vi "SettleDrift_v2.vi"() -> ()   [LabVIEW 2014]
uses:
  shared/CorrelImages (SubVI)Single.vi
  <userlib>/Nanonis Prog Interface V5/Nanonis Prog Interface.lvlib
panel:
  in  "stop":bool
  out "x drift":sgl format="%#_6p"
  out "y drift":sgl format="%#_6p"
  out "y Drift":sgl(graph)
  out "X Drift":sgl(graph)
  in  "Drift correction Pixels":i32=256
  in  "Img Current":sgl=2.5e-11 format="%#_6p"
  in  "Img Bias (V)":sgl=0.02 format="%_2p"
  in  "Img Speed":sgl=3e-08 format="%#_6p"
  in  "Channel index (0-23)":u8(ring) items=["Current"=0, "Z (m)"=14]
  # "Turn continuous scan off"
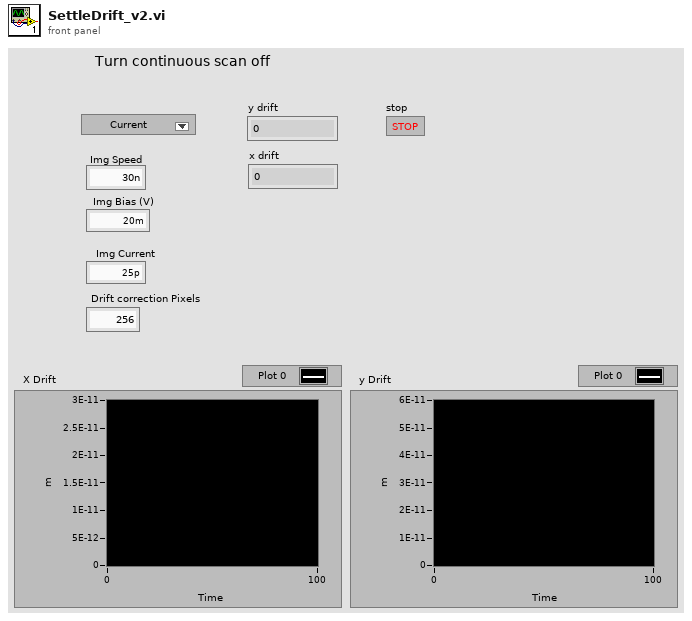
[diagram p1: front panel]
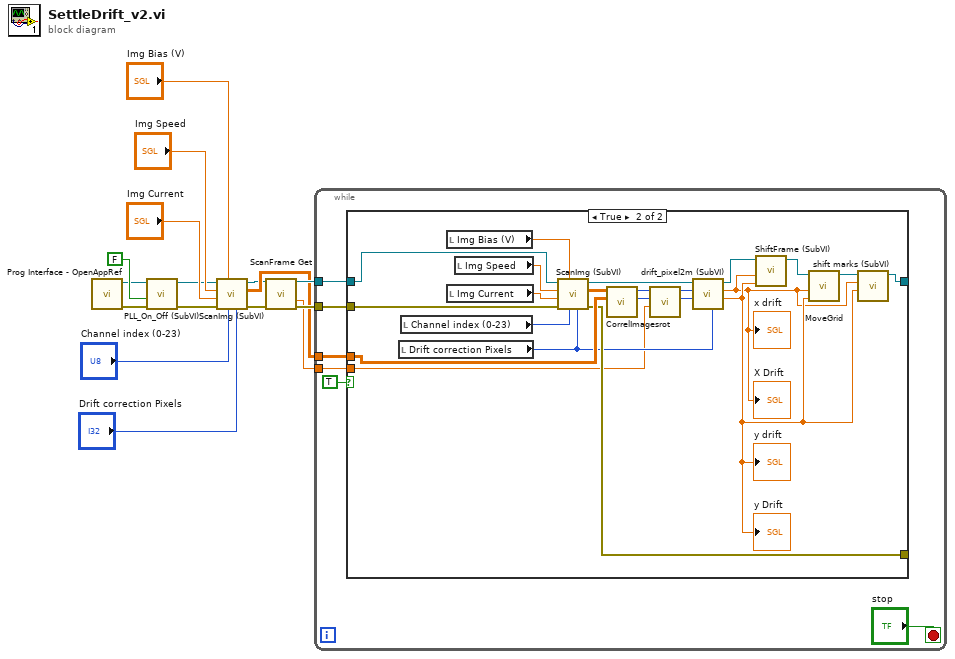
[diagram p0: block diagram]
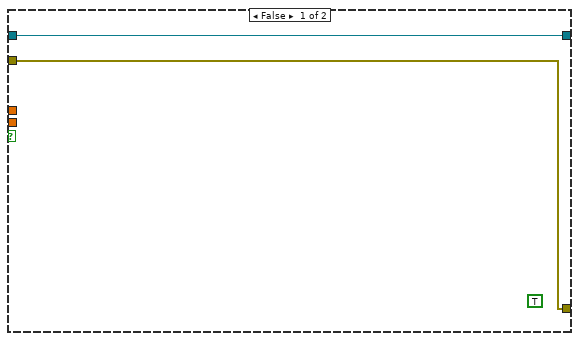
[diagram p2: hidden frame]
diagram:
  n1 = call <userlib>:"Prog Interface - OpenAppRef.vi"() -> ("Error out"=w1:errorcluster, "Application reference"=w2:refnum<vi>)  [unwired: 6 in]
  n2 = call "PLL_On_Off (SubVI).vi"("error in (no error)"=w1, "Output ON/OFF (F=OFF)"=FALSE, "Application in"=w2) -> ("error out"=w7:errorcluster, "Application out"=w8:refnum<vi>)  [unwired: 7 in]
  n3 = call "ScanImg (SubVI).vi"("pixel"="Drift correction Pixels", "Channel index (0-23)"="Channel index (0-23)", "Bias (V)"="Img Bias (V)", "error in (no error)"=w7, "Current"="Img Current", "Img Speed"="Img Speed", "Application in"=w8) -> ("error out"=w3:errorcluster, "Img"=w14:dbl[][], "Application out"=w4:refnum<vi>)  [unwired: 2 in]
  n4 = call <userlib>:"ScanFrame Get.vi"("Application ref in"=w4, "error in (no error)"=w3) -> ("Application ref out"=w16:refnum<vi>, "Angle (deg)"=w13:sgl, "error out"=w15:errorcluster)  [unwired: 9 in, 2 out]
  n5 = while {
    tunnel: w16 -> [w22]
    tunnel: w15 -> [w21]
    tunnel: w14 -> [w20]
    tunnel: w13 -> [w19]
    stop <- "stop" stop-if-true
    n6 = case shown="True" TRUE {
      tunnel: w20 -> [_ w46]
      tunnel: w22 -> [w23 w30]
      tunnel: w21 -> [w24 w45]
      tunnel: [w24 w44] -> _
      tunnel: [w23 w27] -> _
      tunnel: w19 -> [_ w35]
      frame False {
        (unwired) TRUE ("DC active")
      }
      frame True {
        n7 = local read "Drift correction Pixels"() -> (w36:i32)
        n8 = local read "Channel index (0-23)"() -> (w39:u8)
        n9 = local read "Img Bias (V)"() -> (w40:sgl)
        n10 = local read "Img Current"() -> (w41:sgl)
        n11 = local read "Img Speed"() -> (w42:sgl)
        n12 = call "ScanImg (SubVI).vi"("pixel"=w36, "Channel index (0-23)"=w39, "Bias (V)"=w40, "error in (no error)"=w45, "Current"=w41, "Img Speed"=w42, "Application in"=w30) -> ("error out"=w44:errorcluster, "Img"=w43:dbl[][], "Application out"=w37:refnum<vi>)  [unwired: 2 in]
        n13 = call-poly "CorrelImages.vi"("Ref Array"=w46, "New Image"=w43) -> ("Y drift"=w32:i32, "X drift"=w34:i32)  [unwired: 6 in, 2 out]
        n14 = call "rot.vi"("angle"=w35, "y"=w32, "x"=w34) -> ("y'"=w31:i32, "x'"=w33:i32)  [unwired: 7 in]
        n15 = call "drift_pixel2m (SubVI).vi"("Application in"=w37, "X drift"=w33, "Y drift"=w31, "Drift correction Pixels"=w36) -> ("Application out"=w38:refnum<vi>, "x drift"=w25:sgl, "y drift"=w26:sgl)  [unwired: 2 in, 1 out]
        "X Drift" <- w25
        "y Drift" <- w26
        "y drift" <- w26
        "x drift" <- w25
        n16 = call "ShiftFrame (SubVI).vi"("Y shift"=w26, "X shift"=w25, "Application in"=w38) -> ("Application out"=w29:refnum<vi>)  [unwired: 8 in]
        n17 = call "MoveGrid.vi"("y"=w26, "x"=w25, "Application ref in"=w29) -> ("Application ref out"=w28:refnum<vi>)  [unwired: 7 in, 1 out]
        n18 = call "shift marks (SubVI).vi"("y"=w26, "x"=w25, "Application in"=w28) -> ("Application out"=w27:refnum<vi>)  [unwired: 7 in, 1 out]
      }
    }
  }
